vi "Dispose.vi"(8 "error in":errorcluster, 11 "ChicagoStyleCheesePizza":refnum<class "ChicagoStyleCheesePizza.lvclass">) -> (0 "error out":errorcluster)   [LabVIEW 2020, in "FactoryMethod.lvlib" / "PizzaFactoryMethod.lvlib" / "ChicagoStyleCheesePizza.lvclass"]
uses:
  ChicagoStyleCheesePizza.lvclass
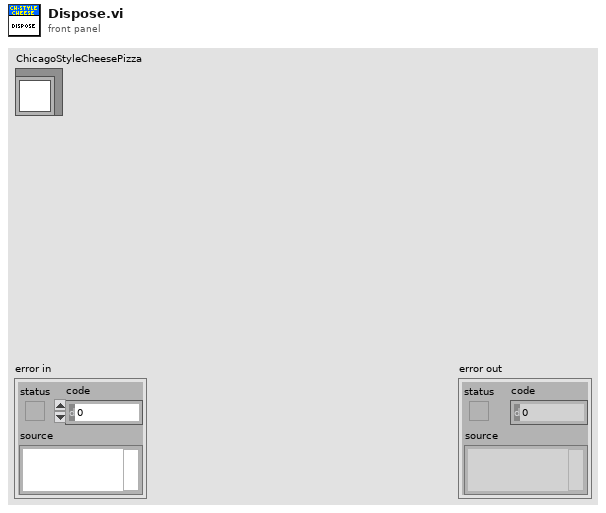
[diagram p1: front panel]
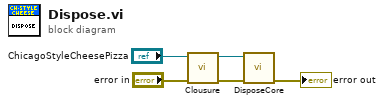
[diagram p0: block diagram]
diagram:
  n1 = call-dynamic "Clousure.vi"("error in"="error in", "ChicagoStyleCheesePizza"="ChicagoStyleCheesePizza") -> ("error out"=w3:errorcluster, "ChicagoStyleCheesePizza"=w4:refnum<class "ChicagoStyleCheesePizza.lvclass">)  [unwired: 8 in]
  n2 = call-dynamic "DisposeCore.vi"("error in (no error)"=w3, "ChicagoStyleCheesePizza"=w4) -> ("error out"=→"error out":errorcluster)  [unwired: 8 in, 1 out]
